vi "Write Fgen Channel.vi"(8 "error in (no error)":errorcluster, 10 "Fgen Channel Setting":T1={"Trgger Type"="Immediate", "Duty Cycle"=0.0, "Amplitude"=1.0, "Frequency"=10000.0, "Output Shape"="Sine Wave", "Phase"=0.0} {"Duty Cycle" format="%#_6f"; "Frequency" format="%#_6p"; "Amplitude" format="%#_6f"}, 11 "Fgen Channel configuration":refnum<class "Fgen Channel configuration.lvclass">) -> (0 "error out":errorcluster, 3 "Fgen Channel configuration out":refnum<class "Fgen Channel configuration.lvclass">)   [LabVIEW 2025, in "Fgen.lvlib" / "Fgen Channel configuration.lvclass"]
uses:
  Fgen Channel configuration.lvclass
  Fgen Channel Setting.ctl
  Fgen Channel configuration.lvclass/Fgen Channel configuration.ctl
panel:
  # "Standard only"
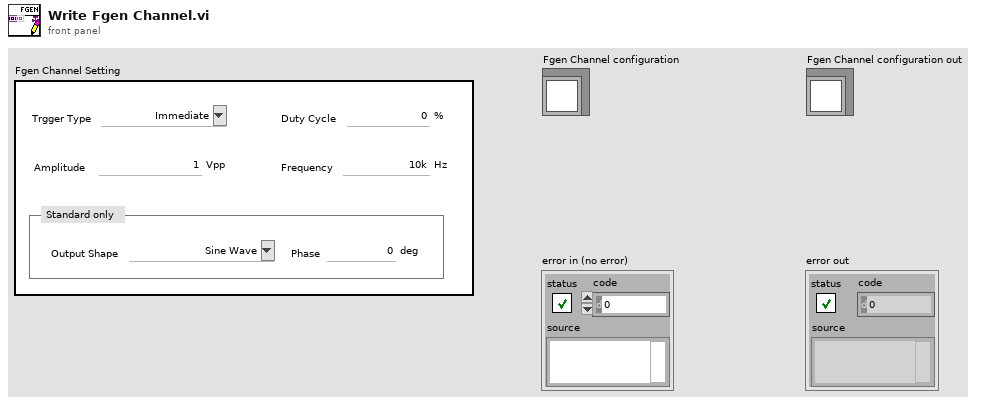
[diagram p1: front panel]
types:
  T1 = typedef "Fgen.lvlib/Fgen Channel configuration.lvclass/Fgen Channel Setting.ctl" = cluster{"Trgger Type":string, "Duty Cycle":dbl, "Amplitude":dbl, "Frequency":dbl, "Output Shape":string, "Phase":dbl}
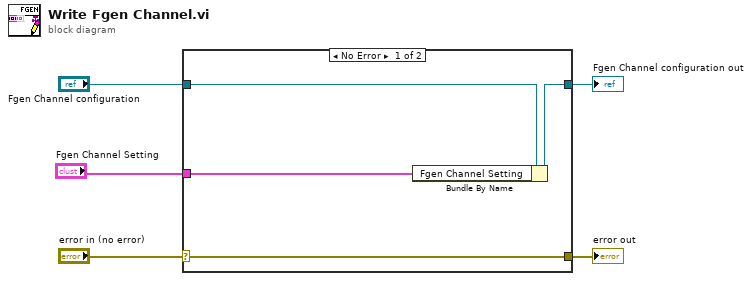
[diagram p0: block diagram]
diagram:
  n1 = case shown="No Error" "error in (no error)" {
    selector: "error in (no error)" -> [w9 w10]
    tunnel: [w9 w10] -> w4
    tunnel: [w7 w11] -> w3
    tunnel: "Fgen Channel configuration" -> [w8 w11]
    tunnel: "Fgen Channel Setting" -> [w6 _]
    frame No Error {
      n2 = Bundle By Name(cluster=w8, "Fgen Channel Setting"=w6) -> (w7:refnum<class "Fgen Channel configuration.lvclass">)
    }
    frame Error {
    }
  }
  "error out" <- w4
  "Fgen Channel configuration out" <- w3
